vi "Report.GenerateChannels.vi"(8 "error in (no error)":errorcluster, 10 "Channel":string, 11 "Properties":variant) -> (0 "error out":errorcluster, 3 "Reports":string[][](array[string]))   [LabVIEW 2015, in "NIAnalysis.lvlib"]
uses:
  NIAnalysis.lvlib
  Types/PropertyGroups.ctl
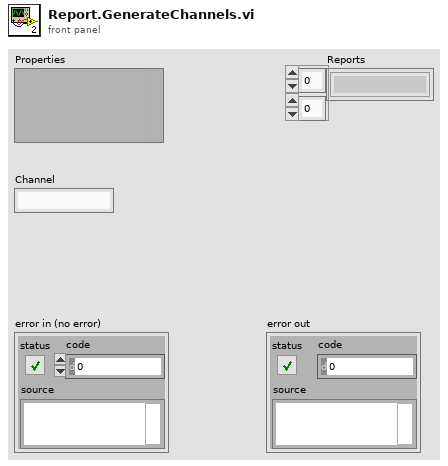
[diagram p1: front panel]
types:
  T1 = typedef "NIAnalysis.lvlib/PropertyGroups.ctl" = cluster{"Pass":bool, "Additional Info":variant}
  T2 = typedef "Type Descriptor Enumeration__ogtk.ctl" = enum8{"<Null>", "I8", "I16", "I32", "I64", "U8", "U16", "U32", "U64", "SGL", "DBL", "EXT", "CSG", "CDB", "CXT", "0x0F", "0x10", "0x11", "0x12", "0x13", "0x14", "Enum U8", "Enum U16", "Enum U32", "Enum U64", "SGL PQ", "DBL PQ", "EXT PQ", "CSG PQ", "CDB PQ", "CXT PQ", "0x1F", "0x20", "Boolean", "0x22", "0x23", "0x24", "0x25", "0x26", "0x27", "0x28", "0x29", "0x2A", "0x2B", "0x2C", "0x2D", "0x2E", "0x2F", "String", "0x31", "Path", "Pict", "0x34", "0x35", "0x36", "DAQ", "0x38", "0x39", "0x3A", "0x3B", "0x3C", "0x3D", "0x3E", "0x3F", "Array", "0x41", "0x42", "0x43", "0x44", "0x45", "0x46", "0x47", "0x48", "0x49", "0x4A", "0x4B", "0x4C", "0x4D", "0x4E", "0x4F", "Cluster", "0x51", "0x52", "Variant", "Waveform", "0x55", "0x56", "0x57", "0x58", "0x59", "0x5A", "0x5B", "0x5C", "0x5D", "0x5E", "0x5F", "0x60", "0x61", "0x62", "0x63", "0x64", "0x65", "0x66", "0x67", "0x68", "0x69", "0x6A", "0x6B", "0x6C", "0x6D", "0x6E", "0x6F", "Refnum"}
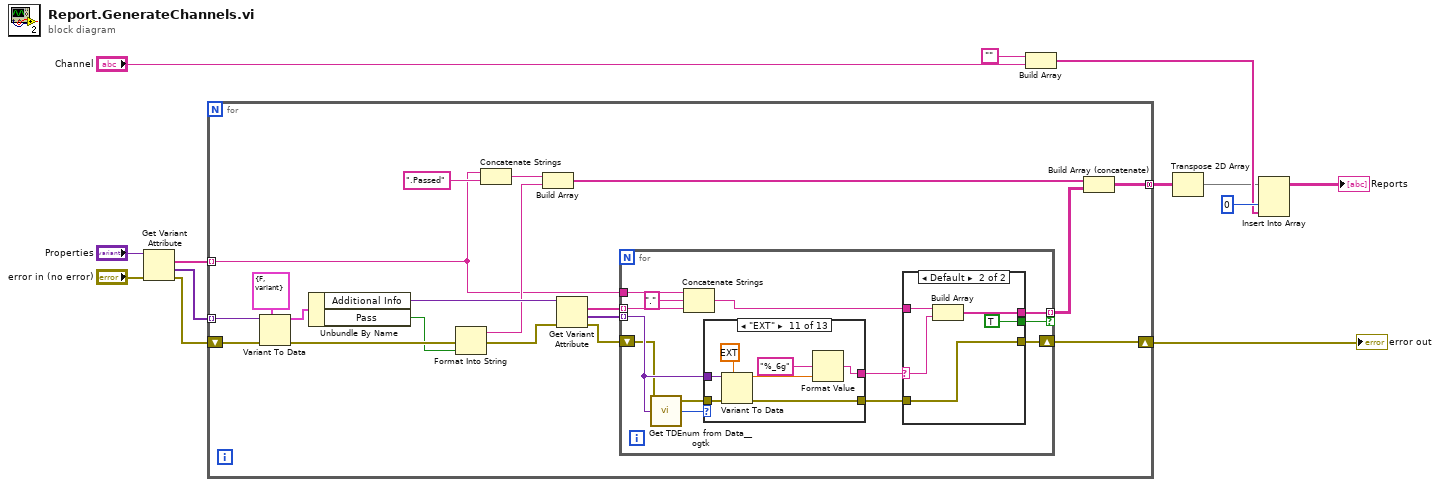
[diagram p0: block diagram]
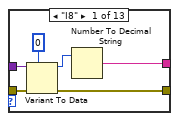
[diagram p3: hidden frame]
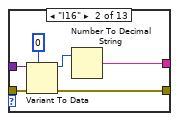
[diagram p4: hidden frame]
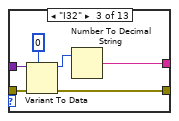
[diagram p5: hidden frame]
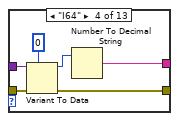
[diagram p6: hidden frame]
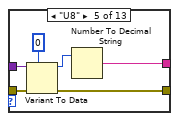
[diagram p7: hidden frame]
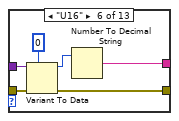
[diagram p8: hidden frame]
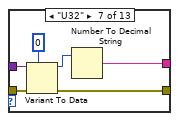
[diagram p9: hidden frame]
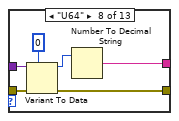
[diagram p10: hidden frame]
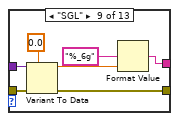
[diagram p11: hidden frame]
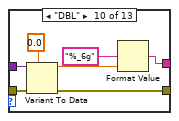
[diagram p12: hidden frame]
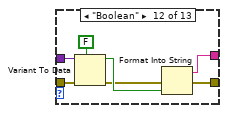
[diagram p13: hidden frame]
diagram:
  n1 = Get Variant Attribute(Variant="Properties", error in="error in (no error)") -> (names=w12:string[], values=w11:variant[], error out=w10:errorcluster)  [unwired: 2 in, 1 out]
  n2 = for {
    shift-right: [w27] -> w8
    shift-left: w10 -> [w29]
    tunnel: w11 -> [w31] mode=indexing
    tunnel: w12 -> [w14] mode=indexing
    tunnel: [w17] -> w4 mode=concatenating
    n3 = Variant To Data(error in=w29, type=T1 {"Pass"=FALSE, "Additional Info"=variant}, Variant=w31) -> (data=w30:T1, error out=w23:errorcluster)
    n4 = Unbundle By Name(w30) -> ("Additional Info"=w28:variant, "Pass"=w21:bool)
    n5 = Format Into String(error in=w23, w21) -> (resulting string=w20:string, error out=w22:errorcluster)  [unwired: 2 in]
    n6 = Concatenate Strings(w14, ".Passed" ("element")) -> (w15:string)
    n7 = Build Array(w15, w20) -> (w19:string[])
    n8 = Get Variant Attribute(Variant=w28, error in=w22) -> (names=w26:string[], values=w24:variant[], error out=w25:errorcluster)  [unwired: 2 in, 1 out]
    n9 = for {
      tunnel: w26 -> [w34] mode=indexing
      shift-right: [w44] -> w27
      shift-left: w25 -> [w41]
      tunnel: w24 -> [w42] mode=indexing
      tunnel: [w38] -> w18 mode=indexing if=w37
      tunnel: w14 -> [w36]
      n10 = call <userlib>:"Get TDEnum from Data__ogtk.vi"("Data"=w42) -> ("Type Descriptor Enumeration"=w43:T2)  [unwired: 4 in]
      n11 = Concatenate Strings(w36, "." ("string"), w34) -> (w33:string)
      n12 = case shown="\"EXT\"" w43 {
        tunnel: w42 -> [w56 w62 w68 w74 w80 w86 w92 w98 w105 w112 w119 w126 _]
        tunnel: w41 -> [w53 w59 w65 w71 w77 w83 w89 w95 w103 w110 w117 w124 w127]
        tunnel: [w52 w58 w64 w70 w76 w82 w88 w94 w99 w106 w113 w122 _] -> w39
        tunnel: [w51 w57 w63 w69 w75 w81 w87 w93 w102 w109 w116 w120 w127] -> w40
        frame "I8" {
          n13 = Variant To Data(error in=w53, type=i8 0 ("default (0 I32)"), Variant=w56) -> (data=w54:i8, error out=w51:errorcluster)
          n14 = Number To Decimal String(number=w54) -> (decimal integer string=w52:string)  [unwired: 1 in]
        }
        frame "I16" {
          n15 = Variant To Data(error in=w59, type=i16 0 ("default (0 I32)"), Variant=w62) -> (data=w60:i16, error out=w57:errorcluster)
          n16 = Number To Decimal String(number=w60) -> (decimal integer string=w58:string)  [unwired: 1 in]
        }
        frame "I32" {
          n17 = Variant To Data(error in=w65, type=0 ("default (0 I32)"), Variant=w68) -> (data=w66:i32, error out=w63:errorcluster)
          n18 = Number To Decimal String(number=w66) -> (decimal integer string=w64:string)  [unwired: 1 in]
        }
        frame "I64" {
          n19 = Variant To Data(error in=w71, type=i64 0 ("default (0 I32)"), Variant=w74) -> (data=w72:i64, error out=w69:errorcluster)
          n20 = Number To Decimal String(number=w72) -> (decimal integer string=w70:string)  [unwired: 1 in]
        }
        frame "U8" {
          n21 = Variant To Data(error in=w77, type=u8 0 ("default (0 I32)"), Variant=w80) -> (data=w78:u8, error out=w75:errorcluster)
          n22 = Number To Decimal String(number=w78) -> (decimal integer string=w76:string)  [unwired: 1 in]
        }
        frame "U16" {
          n23 = Variant To Data(error in=w83, type=u16 0 ("default (0 I32)"), Variant=w86) -> (data=w84:u16, error out=w81:errorcluster)
          n24 = Number To Decimal String(number=w84) -> (decimal integer string=w82:string)  [unwired: 1 in]
        }
        frame "U32" {
          n25 = Variant To Data(error in=w89, type=u32 0 ("default (0 I32)"), Variant=w92) -> (data=w90:u32, error out=w87:errorcluster)
          n26 = Number To Decimal String(number=w90) -> (decimal integer string=w88:string)  [unwired: 1 in]
        }
        frame "U64" {
          n27 = Variant To Data(error in=w95, type=u64 0 ("default (0 I32)"), Variant=w98) -> (data=w96:u64, error out=w93:errorcluster)
          n28 = Number To Decimal String(number=w96) -> (decimal integer string=w94:string)  [unwired: 1 in]
        }
        frame "SGL" {
          n29 = Variant To Data(error in=w103, type=sgl 0.0 ("default (0 I32)"), Variant=w105) -> (data=w100:sgl, error out=w102:errorcluster)
          n30 = Format Value(format string="%_6g", value (0)=w100) -> (output string=w99:string)  [unwired: 1 in]
        }
        frame "DBL" {
          n31 = Variant To Data(error in=w110, type=0.0 ("default (0 I32)"), Variant=w112) -> (data=w107:dbl, error out=w109:errorcluster)
          n32 = Format Value(format string="%_6g", value (0)=w107) -> (output string=w106:string)  [unwired: 1 in]
        }
        frame "EXT" {
          n33 = Variant To Data(error in=w117, type=ext 0.0 ("default (0 I32)"), Variant=w119) -> (data=w114:ext, error out=w116:errorcluster)
          n34 = Format Value(format string="%_6g", value (0)=w114) -> (output string=w113:string)  [unwired: 1 in]
        }
        frame "Boolean" {
          n35 = Variant To Data(error in=w124, type=FALSE, Variant=w126) -> (data=w123:bool, error out=w121:errorcluster)
          n36 = Format Into String(error in=w121, w123) -> (resulting string=w122:string, error out=w120:errorcluster)  [unwired: 2 in]
        }
        frame Default {
        }
      }
      n37 = case shown="Default" w39 {
        selector: w39 -> [_ w48]
        tunnel: w33 -> [_ w49]
        tunnel: [w45 w50] -> w44
        tunnel: w40 -> [w45 w50]
        tunnel: [_ w47] -> w38
        tunnel: [_ TRUE] -> w37
        frame "" {
        }
        frame Default {
          n38 = Build Array(w49, w48) -> (w47:string[])
        }
      }
    }
    n39 = Build Array (concatenate)(w19, w18) -> (w17:string[][])
  }
  "error out" <- w8
  n40 = Build Array("", "Channel") -> (w2:string[])
  n41 = Transpose 2D Array(2D array=w4) -> (transposed array=w1:string[][])
  n42 = Insert Into Array(array=w1, index (col)=0 ("disabled index (col)"), new element=w2) -> (→"Reports":string[][])  [unwired: 1 in]
